vi "Teach.vi"(0 "Neural Network In":T5={"Weigths"=[], "Last Layer Linear"=TRUE, "Add Bias Inputs"=TRUE, "# Inputs"=0, "# Output Neurons/Outputs"=0, "Inputs Scaling"={"X Scaling Vector"=[], "Y Scaling Vector"=[]}, "Outputs Scaling"={"X Scaling Vector"=[], "Y Scaling Vector"=[]}}, 5 "Teaching Set In":T1[](array[typedef]), 7 "Validation Set In":T1[](array[typedef]), 9 "Termination Settings In":T3={"Max Epocs"=10000, "Error Goal"=10.0, "Max Time (s)"=10.0, "Error Evaluation"=enum."Over Teaching Set"}, 11 "Error In":errorcluster) -> (4 "Neural Network Out":T5={"Weigths"=[], "Last Layer Linear"=TRUE, "Add Bias Inputs"=TRUE, "# Inputs"=0, "# Output Neurons/Outputs"=0, "Inputs Scaling"={"X Scaling Vector"=[], "Y Scaling Vector"=[]}, "Outputs Scaling"={"X Scaling Vector"=[], "Y Scaling Vector"=[]}}, 8 "Solution Found":bool, 10 "Error Trend Out":dbl[](array[numeric]), 15 "Error Out":errorcluster)   [LabVIEW 2013, in "Super Simple Neural Network.lvlib"]
doc: "This VI uses RProp algorithm to teach the neural network based on the teaching and validation sets. This VI also calculates the scaling coeficients based on the input teaching vectors. The scaling coeficients will be used whenever you calculate the response of the network to some input.\n\n<b>Teaching Set In</b> - this is the set of teaching vectors that is the basis of teaching the network. Error evaluated over this network is back propagated through the network and is used to update the weights. This error can also be used to stop the teaching algorithm if it's value is smaller than the target error.\n\n<b>Validation Set In</b> - this set is not used to teach the network, only to stop the algorithm if the error is smaller than the target.\n\n<b>Termination Settings In</b> - this cluster defines the maximum number of iterations of the algorithm, the target error goal, max time after which the algorithm will stop and if the error for stopping the algorithm should be calculated over teaching set, validation set or both.\n\n<b>Error Trend Out</b> - this is an array output that can be displayed on a graph that gives information on number of teaching epochs that passed and how the error changed over the epochs.\n\n<b>Solution Found</b> - this indicator informs the user that a solution to the provided teaching samples has been found and the network is ready to operate correctly. This will be false if the teaching algorithm reaches maximum time or number of teaching iterations."
uses:
  Super Simple Neural Network.lvlib
  Types/Neural Network.ctl
  Types/2D Array.ctl
  Types/Scaling Info.ctl
  Types/Stop Settings.ctl
  Types/Error Evaluation.ctl
  Types/Teaching Vector.ctl
  Types/1D Array.ctl
  Scaling/Min Max Array.vi
  Scaling/Extract Coefs for Network.vi
  Scaling/Scale Teaching Validation Vector.vi
  Teaching/Calculate Response Internal.vi
  Teaching/Backpropagation.vi
  Scaling/MD Select 2D DBL.vi
  Scaling/MD Select 1D DBL.vi
  Scaling/Scale Array.vi
  <vilib>/Analysis/baseanly.llb/A x B.vi
  <vilib>/Analysis/baseanly.llb/A x Vector.vi
  <vilib>/Analysis/baseanly.llb/Outer Product.vi
  <vilib>/Analysis/baseanly.llb/Real Outer Product.vi
  <vilib>/Analysis/Matrix/Numeric/Conversions/Matrix To Array.vi
  <vilib>/Analysis/Matrix/Numeric/Conversions/Matrix To Array - RM.vi
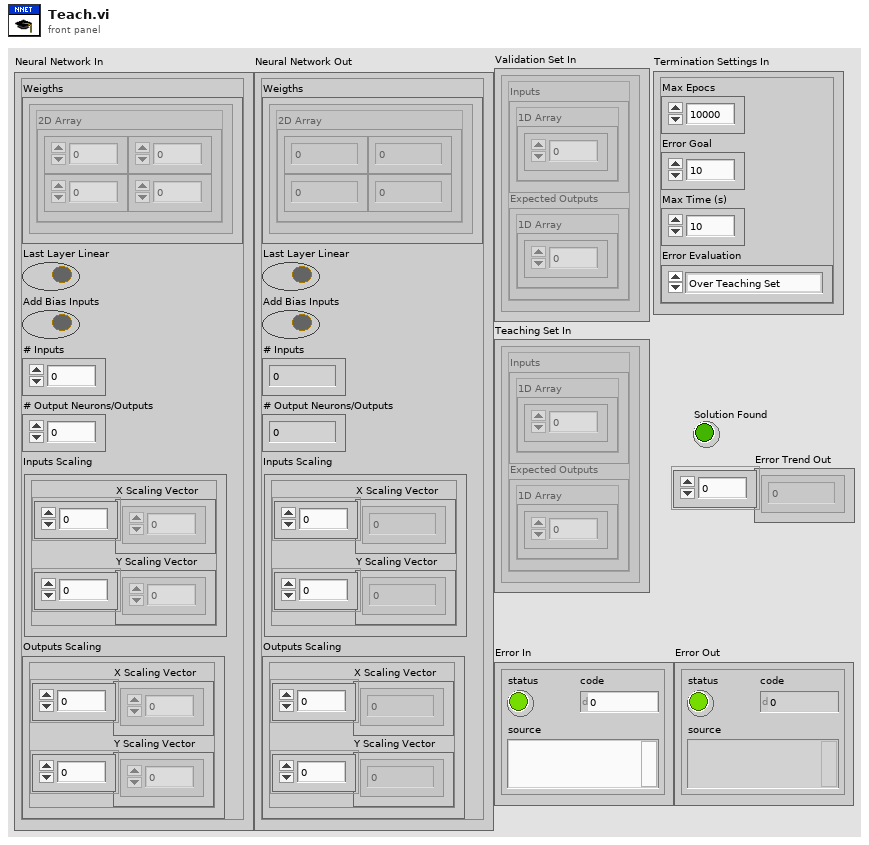
[diagram p1: front panel]
types:
  T1 = typedef "Super Simple Neural Network.lvlib/Teaching Vector.ctl" = cluster{"Inputs":T2, "Expected Outputs":T2}
  T2 = typedef "Super Simple Neural Network.lvlib/1D Array.ctl" = cluster{"1D Array":dbl[]}
  T3 = typedef "Super Simple Neural Network.lvlib/Stop Settings.ctl" = cluster{"Max Epocs":u64, "Error Goal":dbl, "Max Time (s)":dbl, "Error Evaluation":T4}
  T4 = typedef "Super Simple Neural Network.lvlib/Error Evaluation.ctl" = enum16{"Over Both Sets", "Over Validation Set", "Over Teaching Set"}
  T5 = typedef "Super Simple Neural Network.lvlib/Neural Network.ctl" = cluster{"Weigths":T6[], "Last Layer Linear":bool, "Add Bias Inputs":bool, "# Inputs":u32, "# Output Neurons/Outputs":u32, "Inputs Scaling":T7, "Outputs Scaling":T7}
  T6 = typedef "Super Simple Neural Network.lvlib/2D Array.ctl" = cluster{"2D Array":dbl[][]}
  T7 = typedef "Super Simple Neural Network.lvlib/Scaling Info.ctl" = cluster{"X Scaling Vector":dbl[], "Y Scaling Vector":dbl[]}
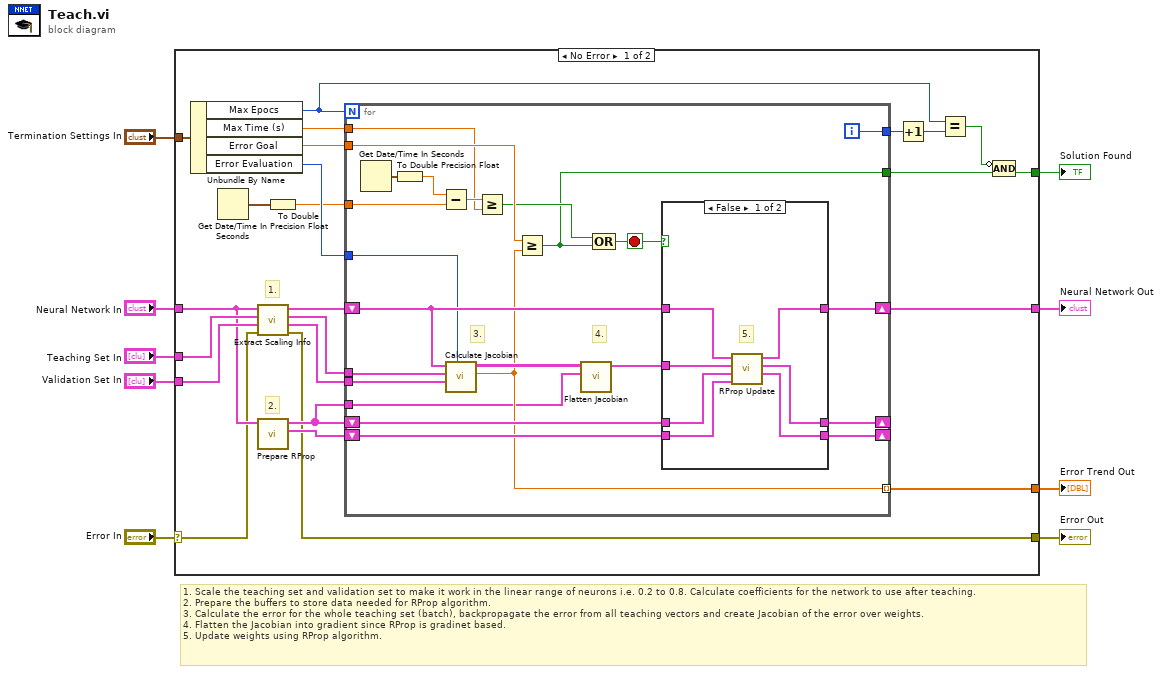
[diagram p0: block diagram]
diagram:
  # "1. Scale the teaching set and validation set to make it work in the linear range of neurons i.e. 0.2 to 0.8. Calculate coefficients for the network to use after teaching.\n2. Prepare the buffers to store data needed for RProp algorithm.\n3. Calculate the error for the whole teaching set (batch), backpropagate the error from all teaching vectors and create Jacobian of the error over weights.\n4. Flatten the Jacobian into gradient since RProp is gradinet based.\n5. Update weights using RProp algorithm."
  n1 = case shown="No Error" "Error In" {
    selector: "Error In" -> [w11 _]
    tunnel: "Teaching Set In" -> [w20 _]
    tunnel: "Validation Set In" -> [w19 _]
    tunnel: "Neural Network In" -> [w16 w67]
    tunnel: "Termination Settings In" -> [w32 _]
    tunnel: [w12 w67] -> w5
    tunnel: [w28 _] -> w4
    tunnel: [w14 _] -> w3
    tunnel: [w10 _] -> w1
    frame No Error {
      # "2."
      # "1."
      n2 = Unbundle By Name(w32) -> ("Max Epocs"=w23:u64, "Max Time (s)"=w30:dbl, "Error Goal"=w29:dbl, "Error Evaluation"=w31:T4)
      n3 = Get Date/Time In Seconds() -> (seconds since 1Jan1904=w27:timestamp)
      n4 = call "Extract Scaling Info.vi"("Error In"=w11, "Validation Set In"=w19, "Teaching Set In"=w20, "Neural Network In"=w16) -> ("Error Out"=w10:errorcluster, "Validation Set Out"=w17:T1[], "Teaching Set Out"=w18:T1[], "Neural Network Out"=w15:T5)  [unwired: 4 in]
      n5 = call "Prepare RProp.vi"("Neural Network In"=w16) -> ("Teach Coef Buffer"=w33:T6[], "Gradient Buffer"=w13:T6[])  [unwired: 9 in]
      n6 = To Double Precision Float(number=w27) -> (double precision float=w26:dbl)
      n7 = for {
        N: w23 -> [_]
        tunnel: w18 -> [w54]
        tunnel: w17 -> [w53]
        shift-right: [w55] -> _
        shift-left: w33 -> [w52]
        shift-right: [w50] -> _
        shift-left: w13 -> [w47]
        shift-right: [w51] -> w12
        shift-left: w15 -> [w49]
        tunnel: w31 -> [w46]
        tunnel: w30 -> [w38]
        tunnel: [w45] -> w28 mode=indexing
        tunnel: w29 -> [w44]
        tunnel: [w35] -> w21
        tunnel: w26 -> [w40]
        tunnel: [w36] -> w25
        tunnel: w13 -> [w34]
        i -> [w36]
        stop <- w43 stop-if-true
        # "4."
        # "3."
        n8 = Get Date/Time In Seconds() -> (seconds since 1Jan1904=w42:timestamp)
        n9 = To Double Precision Float(number=w42) -> (double precision float=w41:dbl)
        n10 = Subtract(x=w41, y=w40) -> (x-y=w39:dbl)
        n11 = call "Calculate Jacobian.vi"("Error Evaluation"=w46, "Validation Set"=w53, "Teaching Set"=w54, "Neural Network In"=w49) -> ("Total Error"=w45:dbl, "Jacobian"=w56:T6[][])  [unwired: 6 in]
        n12 = Greater Or Equal?(x=w39, y=w38) -> (x >= y?=w37:bool)
        n13 = Greater Or Equal?(x=w44, y=w45) -> (x >= y?=w35:bool)
        n14 = call "Flatten Jacobian.vi"("Gradient In"=w34, "Jacobian"=w56) -> ("Gradient Out"=w48:T6[])  [unwired: 9 in]
        n15 = Compound Arithmetic op=OR(w37, w35) -> (w43:bool)
        n16 = case shown="False" w43 {
          tunnel: [w63 w64] -> w55
          tunnel: w52 -> [w62 w64]
          tunnel: [w61 w66] -> w51
          tunnel: [w60 w65] -> w50
          tunnel: w49 -> [w59 w66]
          tunnel: w48 -> [w58 _]
          tunnel: w47 -> [w57 w65]
          frame False {
            # "5."
            n17 = call "RProp Update.vi"("Teaching Coef In"=w62, "Previous Gradient In"=w57, "Current Gradient In"=w58, "Neural Network In"=w59) -> ("Teaching Coef Out"=w63:T6[], "Gradient Out"=w60:T6[], "Neural Network Out"=w61:T5)  [unwired: 5 in]
          }
          frame True {
          }
        }
      }
      n18 = Increment(x=w25) -> (x+1=w24:i32)
      n19 = Equal?(x=w23, y=w24) -> (x = y?=w22:bool)
      n20 = Compound Arithmetic op=AND(invert w22, w21) -> (w14:bool)
    }
    frame Error {
    }
  }
  "Neural Network Out" <- w5
  "Error Out" <- w1
  "Error Trend Out" <- w4
  "Solution Found" <- w3
